vi "Get_Power.vi"(8 "error in":errorcluster, 11 "VISA name":refnum<visa-resource-name>) -> (0 "error out":errorcluster, 1 "valid ?":bool, 2 "Power /W":dbl, 3 "VISA out":refnum<visa-resource-name>)   [LabVIEW 2020]
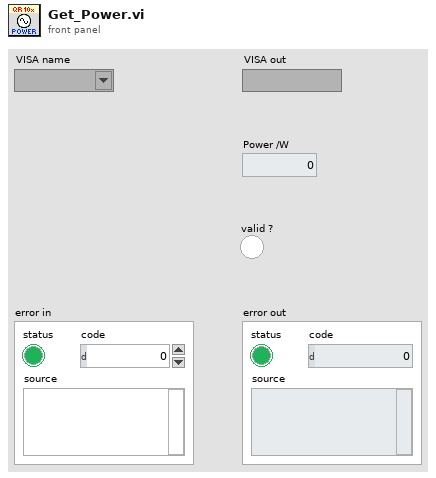
[diagram p1: front panel]
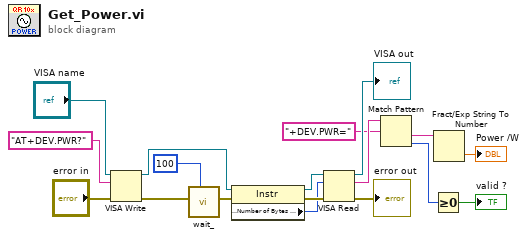
[diagram p0: block diagram]
diagram:
  n1 = VISA Write(VISA resource name="VISA name", write buffer="AT+DEV.PWR?", error in (no error)="error in") -> (VISA resource name out=w14:refnum<visa-resource-name>, error out=w9:errorcluster)  [unwired: 1 out]
  n2 = call "wait_.vi"("milliseconds to wait"=u32 100, "error in"=w9) -> ("error out"=w8:errorcluster)  [unwired: 9 in]
  n3 = property class="Instr"(reference=w14, error in=w8) -> (reference out=w10:refnum<visa-resource-name>, error out=w12:errorcluster, "Serial Settings:Number of Bytes at Serial Port"=w11:u32)
  n4 = VISA Read(VISA resource name=w10, byte count=w11, error in (no error)=w12) -> (VISA resource name out=→"VISA out":refnum<visa-resource-name>, read buffer=w6:string, error out=→"error out":errorcluster)  [unwired: 1 out]
  n5 = Match Pattern(string=w6, regular expression="+DEV.PWR=") -> (after substring=w4:string, offset past match=w2:i32)  [unwired: 1 in, 2 out]
  n6 = Greater Or Equal To 0?(x=w2) -> (x >= 0?=→"valid ?":bool)
  n7 = Fract/Exp String To Number(string=w4) -> (number=→"Power /W":dbl)  [unwired: 3 in, 1 out]
